vi "Acquire.vi"(0 "DAQmx Container In":T1, 1 "Unprocessed Data":refnum<queue>, 3 "error in (no error)":errorcluster) -> (7 "DAQmx Container Out":T1, 10 "error out":errorcluster)   [LabVIEW 2024]
doc: "Perform the acquisition. Replace the contents of this diagram with calls to acquisition hardware."
uses:
  support/Control/Waveform Data Constant.ctl
  support/Control/DAQmx Container.ctl
  <vilib>/DAQmx/read.llb/DAQmx Read (Analog 1D Wfm NChan NSamp).vi
  <vilib>/DAQmx/read.llb/DAQmx Read (Digital 1D Wfm NChan NSamp).vi
  <vilib>/DAQmx/miscellaneous.llb/DAQmx Fill In Error Info.vi
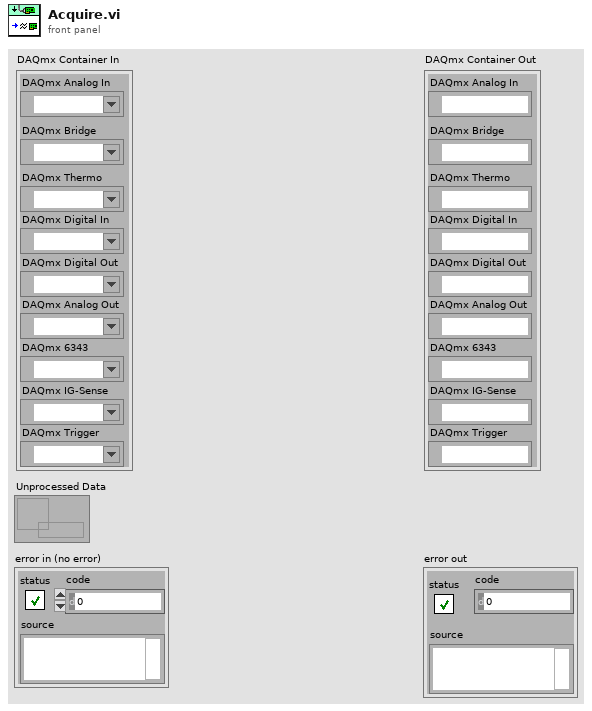
[diagram p1: front panel]
types:
  T1 = typedef "DAQmx Container.ctl" = cluster{"DAQmx Analog In":refnum<k21>, "DAQmx Digital In":refnum<k21>, "DAQmx Digital Out":refnum<k21>, "DAQmx Analog Out":refnum<k21>, "DAQmx 6343":refnum<k21>, "DAQmx IG-Sense":refnum<k21>, "DAQmx Thermo":refnum<k21>, "DAQmx Bridge":refnum<k21>, "DAQmx Trigger":refnum<k21>}
  T2 = typedef "Waveform Data Constant.ctl" = cluster{"AI":waveform(dbl)[], "TC":waveform(dbl)[], "BC":waveform(dbl)[], "DI":digitalwaveform[], "DI2":digitalwaveform[]}
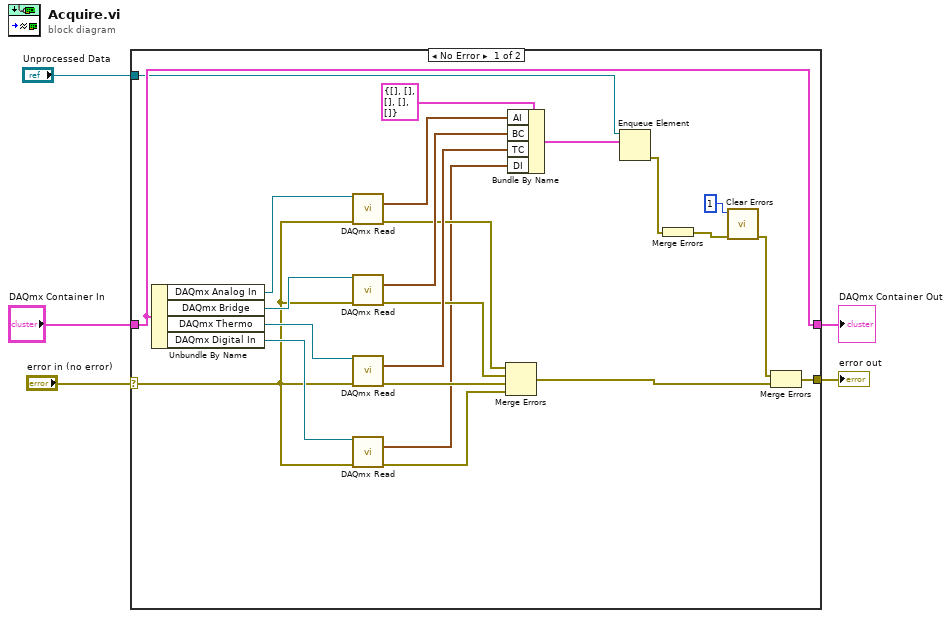
[diagram p0: block diagram]
diagram:
  n1 = case shown="No Error" "error in (no error)" {
    selector: "error in (no error)" -> [w11 w29]
    tunnel: [w28 w29] -> w4
    tunnel: "DAQmx Container In" -> [w27 w30]
    tunnel: [w27 w30] -> w1
    tunnel: "Unprocessed Data" -> [w22 _]
    frame No Error {
      n2 = Unbundle By Name(w27) -> ("DAQmx Analog In"=w26:refnum<k21>, "DAQmx Bridge"=w21:refnum<k21>, "DAQmx Thermo"=w25:refnum<k21>, "DAQmx Digital In"=w24:refnum<k21>)
      n3 = call-poly <vilib>:"DAQmx Read.vi"("task/channels in"=w26, "error in"=w11) -> ("data"=w6:waveform(dbl)[], "error out"=w17:errorcluster)  [unwired: 11 in, 1 out]
      n4 = call-poly <vilib>:"DAQmx Read.vi"("task/channels in"=w21, "error in"=w11) -> ("data"=w20:waveform(dbl)[], "error out"=w16:errorcluster)  [unwired: 11 in, 1 out]
      n5 = call-poly <vilib>:"DAQmx Read.vi"("task/channels in"=w25, "error in"=w11) -> ("data"=w19:waveform(dbl)[], "error out"=w15:errorcluster)  [unwired: 11 in, 1 out]
      n6 = call-poly <vilib>:"DAQmx Read.vi"("task/channels in"=w24, "error in"=w11) -> ("data"=w9:digitalwaveform[], "error out"=w14:errorcluster)  [unwired: 11 in, 1 out]
      n7 = Merge Errors(w17, w16, w15, w14) -> (w18:errorcluster)
      n8 = Bundle By Name(cluster=T2 {"AI"=[], "TC"=[], "BC"=[], "DI"=[], "DI2"=[]} ("Data Constant"), "AI"=w6, "BC"=w20, "TC"=w19, "DI"=w9) -> (w23:T2)
      n9 = Enqueue Element(queue=w22, element=w23) -> (error out=w7:errorcluster)  [unwired: 2 in, 2 out]
      n10 = Merge Errors(w7) -> (w8:errorcluster)
      n11 = call <vilib>:"Clear Errors.vi"("error in (no error)"=w8, "specific error code to clear (0: all)"=1) -> ("error out"=w12:errorcluster)  [unwired: 4 in, 1 out]
      n12 = Merge Errors(w12, w18) -> (w28:errorcluster)
    }
    frame Error {
    }
  }
  "error out" <- w4
  "DAQmx Container Out" <- w1
